vi "Write Version.vi"(9 "Version string":string, 10 "Version":T1, 11 "ProjectItem in":refnum<class "ProjectItem.lvclass">) -> (3 "ProjectItem out":refnum<class "ProjectItem.lvclass">)   [LabVIEW 2019, in "SolutionBuilder.lvlib" / "ProjectItem.lvclass"]
uses:
  ProjectItem.lvclass
  Community/slnbld_BuildSpecVersion.ctl
  ProjectItem.lvclass/ProjectItem.ctl
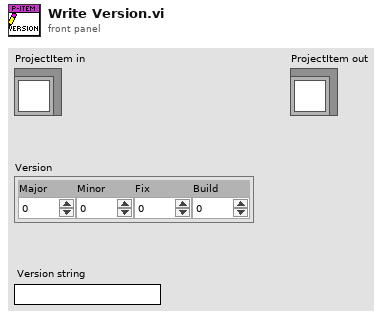
[diagram p1: front panel]
types:
  T1 = typedef "SolutionBuilder.lvlib/ProjectItem.lvclass/slnbld_BuildSpecVersion.ctl" = cluster{"Major":u16, "Minor":u16, "Fix":u16, "Build":u16}
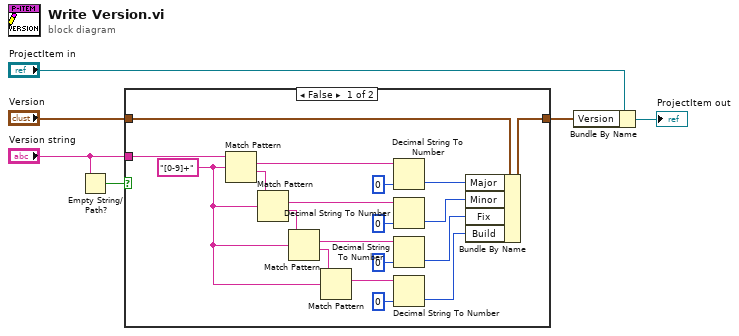
[diagram p0: block diagram]
diagram:
  n1 = Empty String/Path?(string/path="Version string") -> (empty?=w1:bool)
  n2 = case shown="False" w1 {
    tunnel: "Version" -> [w17 w26]
    tunnel: [w12 w26] -> w3
    tunnel: "Version string" -> [w11 _]
    frame False {
      w22 = "[0-9]+" ("regular expression")
      n3 = Match Pattern(string=w11, regular expression=w22) -> (match substring=w21:string, after substring=w25:string)  [unwired: 1 in, 2 out]
      n4 = Match Pattern(string=w25, regular expression=w22) -> (match substring=w20:string, after substring=w24:string)  [unwired: 1 in, 2 out]
      n5 = Match Pattern(string=w24, regular expression=w22) -> (match substring=w19:string, after substring=w23:string)  [unwired: 1 in, 2 out]
      n6 = Match Pattern(string=w23, regular expression=w22) -> (match substring=w18:string)  [unwired: 1 in, 3 out]
      n7 = Decimal String To Number(string=w21, default (0L)=u16 0 ("default (0 I32)")) -> (number=w16:u16)  [unwired: 1 in, 1 out]
      n8 = Decimal String To Number(string=w20, default (0L)=u16 0 ("default (0 I32)")) -> (number=w15:u16)  [unwired: 1 in, 1 out]
      n9 = Decimal String To Number(string=w19, default (0L)=u16 0 ("default (0 I32)")) -> (number=w14:u16)  [unwired: 1 in, 1 out]
      n10 = Decimal String To Number(string=w18, default (0L)=u16 0 ("default (0 I32)")) -> (number=w13:u16)  [unwired: 1 in, 1 out]
      n11 = Bundle By Name(cluster=w17, "Major"=w16, "Minor"=w15, "Fix"=w14, "Build"=w13) -> (w12:T1)
    }
    frame True {
    }
  }
  n12 = Bundle By Name(cluster="ProjectItem in", "Version"=w3) -> (→"ProjectItem out":refnum<class "ProjectItem.lvclass">)
